vi "Escrever Log.vi"(6 "Priorizar mensagem":bool, 8 "error in (no error)":errorcluster, 9 "Dados para Log":string, 10 "VI":refnum<vi>, 11 "Queue in":refnum<queue>) -> (0 "error out":errorcluster, 3 "dup Message Queue":refnum<queue>)   [LabVIEW 2020]
doc: "Adiciona na fila a mensagem desejada."
uses:
  Message Queue/Message Cluster.ctl
  Message Queue/Enqueue Message (Single).vi
  Message Queue/Message Queue.lvlib
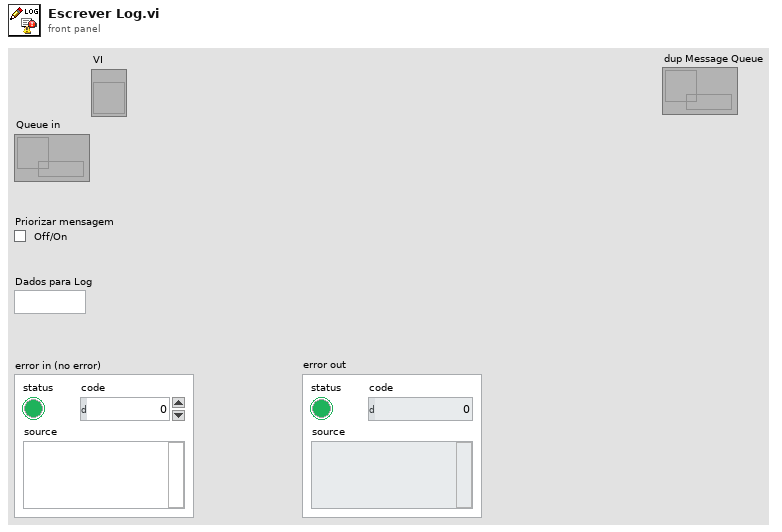
[diagram p1: front panel]
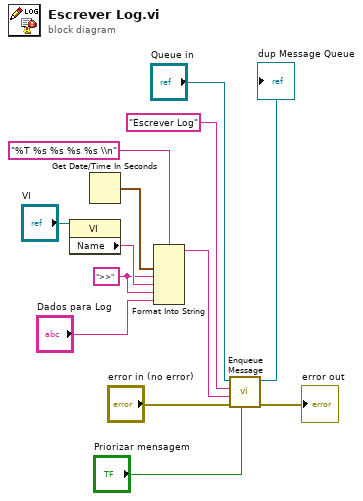
[diagram p0: block diagram]
diagram:
  w5 = ">>" ("input 2")
  n1 = property class="VI"(reference="VI") -> ("Name"=w6:string)  [unwired: 1 in, 2 out]
  n2 = Get Date/Time In Seconds() -> (seconds since 1Jan1904=w8:timestamp)
  n3 = Format Into String(format string="%T %s %s %s %s \\n", w8, w5, w6, w5, "Dados para Log") -> (resulting string=w3:string)  [unwired: 2 in, 1 out]
  n4 = call-poly "Enqueue Message.vi"("Priority Message? (F)"="Priorizar mensagem", "error in (no error)"="error in (no error)", "Message Data"=w3, "Message"="Escrever Log", "Message Queue"="Queue in") -> ("error out"=→"error out":errorcluster, "dup Message Queue"=→"dup Message Queue":refnum<queue>)  [unwired: 5 in]
